vi "HexString to AsciiString.vi"(0 "Hex String":string, 11 "Error In":errorcluster) -> (4 "ASCII String":string, 15 "Error Out":errorcluster)   [LabVIEW 2023]
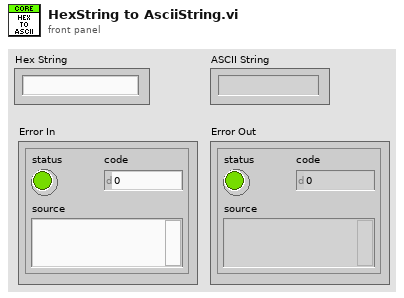
[diagram p1: front panel]
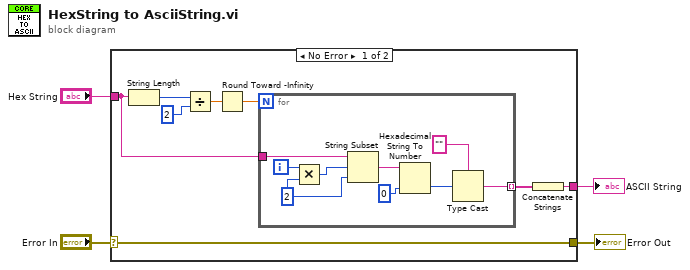
[diagram p0: block diagram]
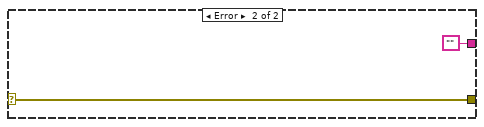
[diagram p2: hidden frame]
diagram:
  n1 = case shown="No Error" "Error In" {
    selector: "Error In" -> [w5 w23]
    tunnel: [w7 ""] -> w4
    tunnel: "Hex String" -> [w6 _]
    tunnel: [w5 w23] -> w1
    frame No Error {
      n2 = String Length(string=w6) -> (length=w12:i32)
      n3 = Divide(x=w12, y=2) -> (x/y=w10:dbl)
      n4 = Round Toward -Infinity(1:w10) -> (0:w9:dbl)
      n5 = for {
        N: w9 -> [_]
        tunnel: w6 -> [w21]
        tunnel: [w13] -> w8 mode=indexing
        i -> [w20]
        w18 = 2 ("length (rest)")
        n6 = Multiply(x=w20, y=w18) -> (x*y=w19:i32)
        n7 = String Subset(string=w21, offset (0)=w19, length (rest)=w18) -> (substring=w17:string)
        n8 = Hexadecimal String To Number(string=w17, default (0uL)=u8 0 ("default (0 U32)")) -> (number=w15:u8)  [unwired: 1 in, 1 out]
        n9 = Type Cast(type="", x=w15) -> (*(type *) &x=w13:string)
      }
      n10 = Concatenate Strings(w8) -> (w7:string)
    }
    frame Error {
    }
  }
  "ASCII String" <- w4
  "Error Out" <- w1
